vi "Actor Core.vi"(8 "error in":errorcluster, 11 "Unit_Test_AFG in":refnum<class "Unit_Test_AFG.lvclass">) -> (0 "error out":errorcluster, 3 "Actor out":refnum<class "Actor.lvclass">)   [LabVIEW 2020, in "Unit_Test_AFG.lvlib" / "Unit_Test_AFG.lvclass"]
doc: "(<B>Filename</B>: Actor Framework.lvlib:Actor.lvclass:Actor Core.vi)\n\nReceives messages to the actor, reacts to them, and initiates any error handling that may shut the actor down.\n\nDescendant classes may override this VI to append parallel tasks for the actor to complete while it handles messages. Overrides use the Call Parent Class Method node."
uses:
  Unit_Test_AFG.lvclass
  C:/Program Files/National Instruments/LabVIEW 2020/vi.lib/ActorFramework/Actor/Actor.lvclass
  <vilib>/ActorFramework/Actor/Actor.lvclass
  Actor_AFG/Actor_AFG/Actor_AFG.lvclass
  Unit_Test_AFG.lvclass/Unit_Test_AFG.ctl
  <vilib>/ActorFramework/Actor/Actor.lvclass/Actor.ctl
  <vilib>/ActorFramework/Message Enqueuer/Message Enqueuer.lvclass/Message Enqueuer.ctl
  <vilib>/ActorFramework/Stop Msg/Stop Msg.lvclass/Stop Msg.ctl
  Actor_AFG/Actor_AFG Messages/Setup Pulse Waveform Msg/Setup Pulse Waveform Msg.lvclass/Setup Pulse Waveform Msg.ctl
  Actor_AFG/Actor_AFG Messages/AFG Setup Cycle Msg/AFG Setup Cycle Msg.lvclass/AFG Setup Cycle Msg.ctl
  Actor_AFG/Actor_AFG Messages/AFG Enable Output Msg/AFG Enable Output Msg.lvclass/AFG Enable Output Msg.ctl
  <vilib>/ActorFramework/Message Enqueuer/Init from Existing Queue.vi
  <vilib>/ActorFramework/Stop Msg/Send Emergency Stop.vi
  <vilib>/ActorFramework/Stop Msg/Send Normal Stop.vi
  <vilib>/ActorFramework/Message Enqueuer/Enqueue.vi
  <vilib>/ActorFramework/Message Enqueuer/Enqueue Critical.vi
  <vilib>/ActorFramework/Stop Msg/Stop Msg.lvclass
  C:/Program Files/National Instruments/LabVIEW 2020/vi.lib/ActorFramework/Message/Message.lvclass
  Actor_AFG/Actor_AFG Messages/Setup Pulse Waveform Msg/Setup Pulse Waveform Msg.lvclass
  Actor_AFG/Actor_AFG Messages/AFG Setup Cycle Msg/AFG Setup Cycle Msg.lvclass
  Actor_AFG/Actor_AFG Messages/AFG Enable Output Msg/AFG Enable Output Msg.lvclass
  <vilib>/ActorFramework/Message Priority Queue/Priority Enqueue.vi
  <vilib>/ActorFramework/Message Enqueuer/Message Enqueuer.lvclass
panel:
  in  "Repeat":bool
  in  "Cycle":i32=1 min=1
  in  "Delay":dbl=50.0
  in  "Spacing":dbl=50.0
  in  "Reset Pulse Conf":T1={"V Conf"={"Bias"=-0.5, "Amp"=-2.5}, "T Conf"={"Rise Time"=5.0, "Fall Time"=5.0, "Pulse Width"=20.0}}
  in  "Set Pulse Conf":T1={"V Conf"={"Bias"=1.0, "Amp"=2.5}, "T Conf"={"Rise Time"=5.0, "Fall Time"=5.0, "Pulse Width"=20.0}}
  in  "Configure Pulse":bool
  in  "Output On/Off":bool
  out "log":string[](array[string])
  # "AFG Unit Test Front Panel"
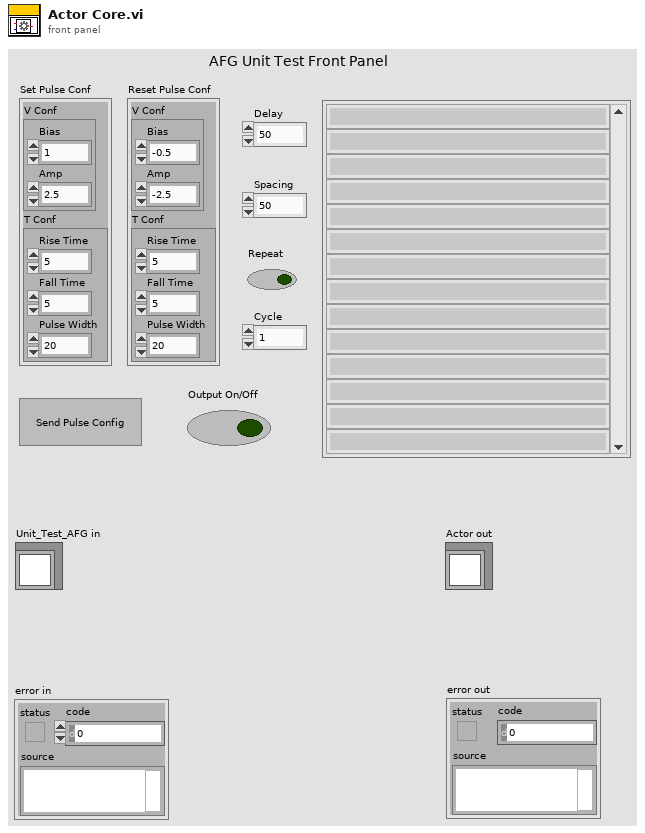
[diagram p1: front panel]
types:
  T1 = cluster{"V Conf":cluster{"Bias":dbl, "Amp":dbl}, "T Conf":cluster{"Rise Time":dbl, "Fall Time":dbl, "Pulse Width":dbl}}
  T2 = enum32{"Invalid", "Standard", "Closed", "Hidden", "Minimized", "Maximized"}
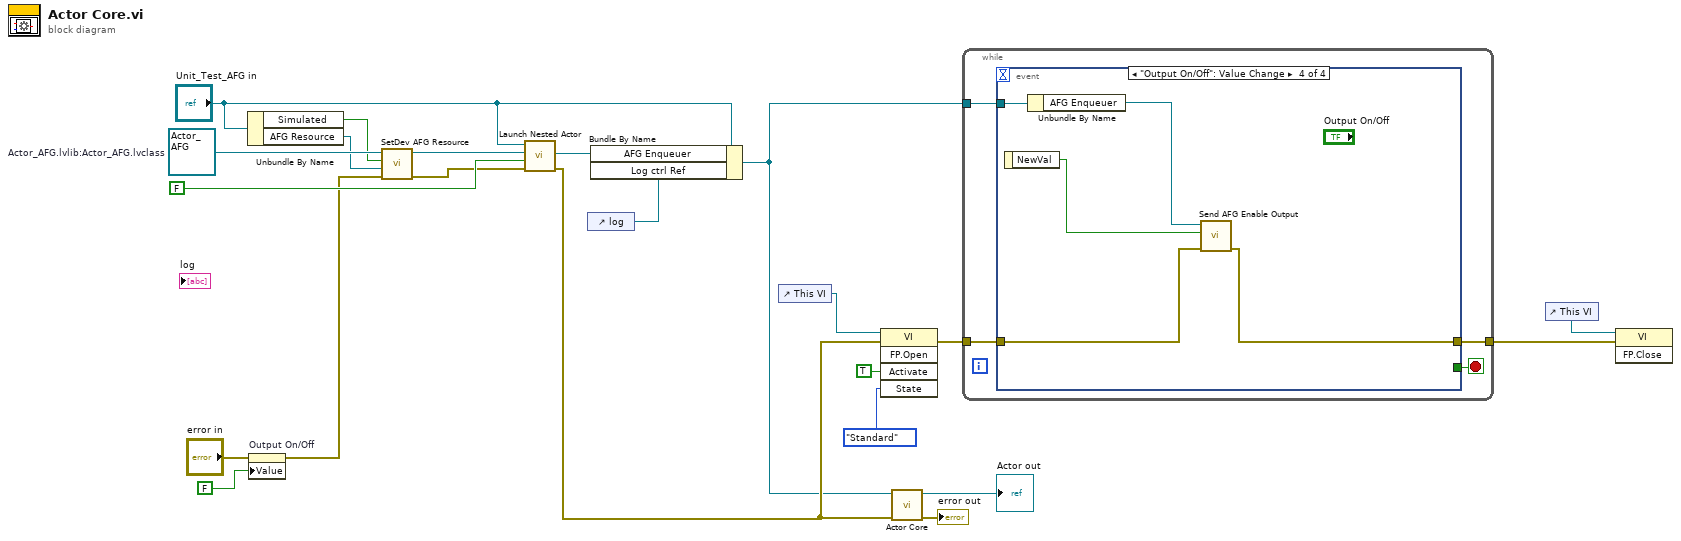
[diagram p0: block diagram]
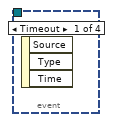
[diagram p2: hidden frame]
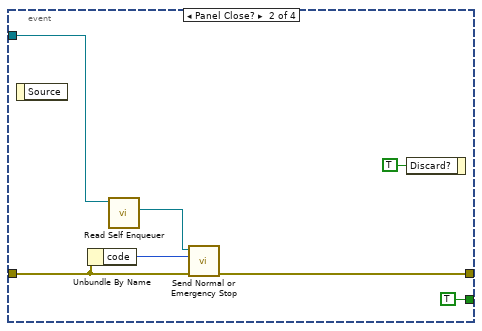
[diagram p3: hidden frame]
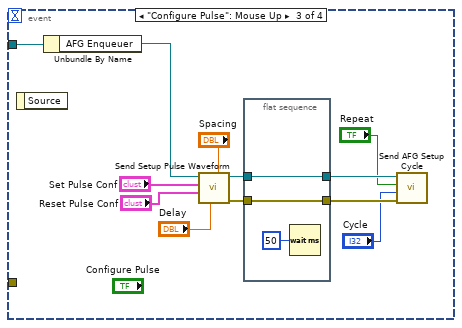
[diagram p4: hidden frame]
diagram:
  w15 = refnum<class "Actor_AFG.lvclass"> refnum  # Actor_AFG.lvlib:Actor_AFG.lvclass
  n1 = Unbundle By Name("Unit_Test_AFG in") -> ("Simulated"=w13:bool, "AFG Resource"=w12:refnum<visa-resource-name>)
  n2 = property on="Output On/Off" class="Bool (strict)"(error in="error in", "Value"=FALSE ("Output On/Off")) -> (error out=w2:errorcluster)  [unwired: 1 in, 1 out]
  n3 = call-dynamic "SetDev AFG Resource.vi"("error in (no error)"=w2, "AFG VISA Addr"=w12, "Simulated"=w13, "Actor_AFG in"=w15) -> ("error out"=w11:errorcluster, "Actor_AFG out"=w14:refnum<class "Actor_AFG.lvclass">)  [unwired: 6 in]
  n4 = call <vilib>:"Launch Nested Actor.vi"("error in (no error)"=w11, "Auto-stop? (T)"=FALSE, "Nested Actor"=w14, "Caller Actor in"="Unit_Test_AFG in") -> ("error out"=w10:errorcluster, "Nested Actor's Enqueuer"=w8:refnum<class "Message Enqueuer.lvclass">)  [unwired: 5 in, 1 out]
  n5 = control-ref of="log"() -> (w4:refnum<vi>)
  n6 = Bundle By Name(cluster="Unit_Test_AFG in", "AFG Enqueuer"=w8, "Log ctrl Ref"=w4) -> (w7:refnum<class "Unit_Test_AFG.lvclass">)
  n7 = control-ref of="This VI"() -> (w20:refnum<vi>)
  n8 = invoke class="VI" method="FP.Open"(reference=w20, error in=w10, "Activate"=TRUE ("Activate?"), "State"=T2."Standard") -> (error out=w17:errorcluster)  [unwired: 1 in, 4 out]
  n9 = call-parent "Actor Core.vi"("error in"=w10, "Actor in"=w7) -> ("error out"=→"error out":errorcluster, "Actor out"=→"Actor out":refnum<class "Actor.lvclass">)  [unwired: 8 in]
  n10 = while {
    tunnel: w17 -> [w24]
    tunnel: w7 -> [w25]
    tunnel: [w23] -> w5
    stop <- w26 stop-if-true
    n11 = event shown="[3] \"Output On/Off\": Value Change" {
      selector: _ -> [_ _ _ _]
      dyn-events: _ -> [_ _ _ _]
      timeout: _ -> [_ _ _ _]
      tunnel: [_ TRUE _ _] -> w26
      tunnel: w25 -> [_ w32 w45 w53]
      tunnel: w24 -> [_ w31 _ w51]
      tunnel: [_ w28 _ w50] -> w23
      event Timeout {
        n12 = event-data() -> ()  [unwired: 1 in, 3 out]
      }
      event Panel Close? {
        n13 = event-data() -> ()  [unwired: 1 in, 1 out]
        n14 = Unbundle By Name(w31) -> ("code"=w30:i32)
        n15 = call <vilib>:"Read Self Enqueuer.vi"("Actor"=w32) -> ("Self Enqueuer"=w29:refnum<class "Message Enqueuer.lvclass">)  [unwired: 10 in]
        n16 = call <vilib>:"Send Normal or Emergency Stop.vi"("error in (no error)"=w31, "final error code"=w30, "Message Enqueuer"=w29) -> ("error out"=w28:errorcluster)  [unwired: 8 in]
        n17 = event-data("Discard?"=TRUE) -> ()  [unwired: 1 in, 1 out]
      }
      event "Configure Pulse": Mouse Up {
        n18 = event-data() -> ()  [unwired: 1 in, 1 out]
        n19 = Unbundle By Name(w45) -> ("AFG Enqueuer"=w44:refnum<class "Message Enqueuer.lvclass">)
        n20 = call "Send Setup Pulse Waveform.vi"("Spacing"="Spacing", "Delay"="Delay", "Reset Pulse Conf"="Reset Pulse Conf", "Set Pulse Conf"="Set Pulse Conf", "Message Enqueuer"=w44) -> ("error out"=w36:errorcluster, "Message Enqueuer out"=w39:refnum<class "Message Enqueuer.lvclass">)  [unwired: 5 in]
        n21 = flat-sequence {
          tunnel: w39 -> [w48]
          tunnel: [w48] -> w38
          tunnel: [w47] -> w37
          tunnel: w36 -> [w47]
          frame #0 {
            n22 = Wait (ms)(milliseconds to wait=u32 50) -> ()  [unwired: 1 out]
          }
        }
        n23 = call "Send AFG Setup Cycle.vi"("error in (no error)"=w37, "Cycles"="Cycle", "Continuous"="Repeat", "Message Enqueuer"=w38) -> ()  [unwired: 6 in, 2 out]
      }
      event "Output On/Off": Value Change {
        n24 = event-data() -> ("NewVal"=w49:bool)  [unwired: 1 in]
        n25 = Unbundle By Name(w53) -> ("AFG Enqueuer"=w52:refnum<class "Message Enqueuer.lvclass">)
        n26 = call "Send AFG Enable Output.vi"("error in (no error)"=w51, "Enable Output (T: Enable)"=w49, "Message Enqueuer"=w52) -> ("error out"=w50:errorcluster)  [unwired: 7 in, 1 out]
      }
    }
  }
  n27 = control-ref of="This VI"() -> (w6:refnum<vi>)
  n28 = invoke class="VI" method="FP.Close"(reference=w6, error in=w5) -> ()  [unwired: 1 in, 3 out]
